vi "test_Export Configuration_Error.vi"(8 "error in (no error)":errorcluster, 11 "TestCase in":refnum<class "FPGA Addon Scripting API Unit Tests.lvclass">=refnum) -> (0 "error out":errorcluster, 3 "TestCase out":refnum<class "FPGA Addon Scripting API Unit Tests.lvclass">)   [LabVIEW 2026, in "FPGA Addon Scripting API Unit Tests.lvclass"]
uses:
  FPGA Addon Scripting API Unit Tests.lvclass
  FPGA Addon Test Class/FPGA Addon Test Class.lvclass
  APIs/Scripting API/Scripting API.lvlib
  APIs/Scripting API/Public/Bitfile Resources/Import Bitfile Scalars (Instances)/Import Scalars - all.vi
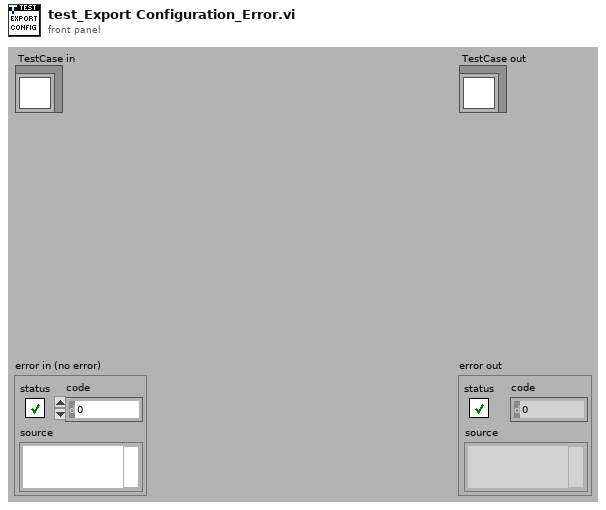
[diagram p1: front panel]
types:
  T1 = typedef "Custom Device API.lvlib/Custom Device Item Ref.ctl" = u64
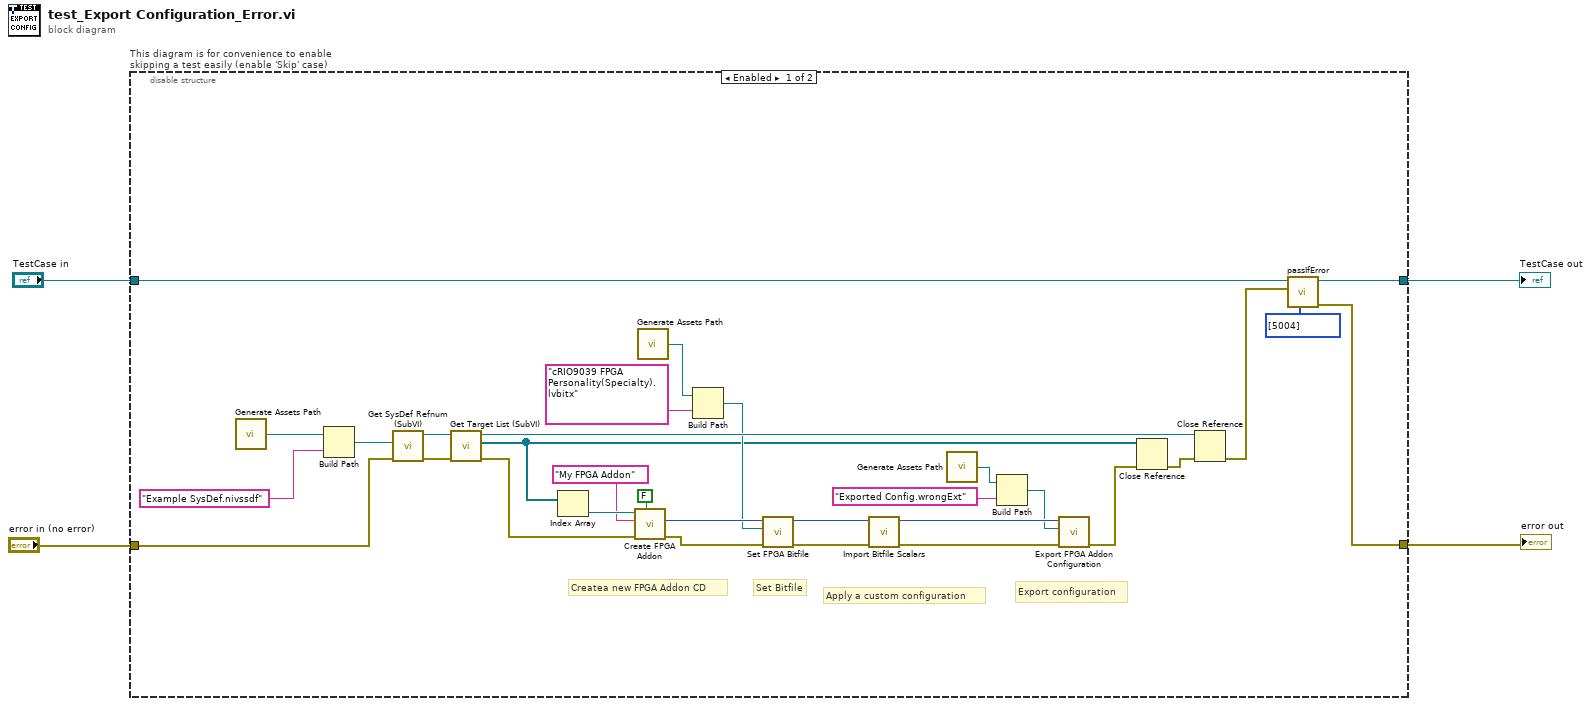
[diagram p0: block diagram]
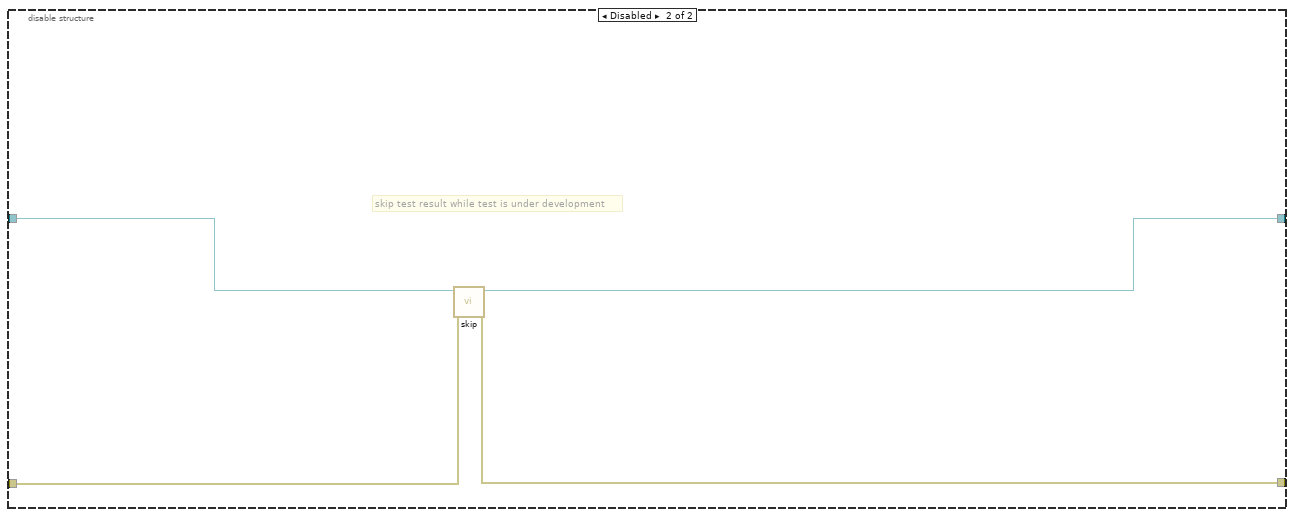
[diagram p2: hidden frame]
diagram:
  n1 = disable-structure "This diagram is for convenience to enable skipping a test easily (enable 'Skip' case)" shown="Enabled" {
    disable-tunnel: "TestCase in" -> [w9 w39]
    disable-tunnel: [w6 w37] -> w1
    disable-tunnel: [w7 w38] -> w3
    disable-tunnel: "error in (no error)" -> [w29 w36]
    frame Enabled {
      # "Export configuration"
      # "Apply a custom configuration"
      # "Set Bitfile"
      # "Createa new FPGA Addon CD"
      n2 = call "Generate Assets Path.vi"() -> ("Assets path"=w35:path)
      n3 = Build Path(base path=w35, name or relative path="Example SysDef.nivssdf") -> (appended path=w33:path)
      n4 = call "Get SysDef Refnum (SubVI).vi"("error in (no error)"=w29, "System Definition path"=w33) -> ("error out"=w28:errorcluster, "NationalInstruments.VeriStand.SystemDefinitionAPI.SystemDefinition"=w32:refnum<k39>)  [unwired: 8 in]
      n5 = call "Get Target List (SubVI).vi"("error in (no error)"=w28, "NationalInstruments.VeriStand.SystemDefinitionAPI.SystemDefinition"=w32) -> ("error out"=w27:errorcluster, "Target List Refnums"=w12:refnum<k39>[], "NationalInstruments.VeriStand.SystemDefinitionAPI.SystemDefinition"=w26:refnum<k39>)  [unwired: 7 in]
      n6 = Index Array(array=w12) -> (element=w31:refnum<k39>)  [unwired: 1 in]
      n7 = call "Create FPGA Addon.vi"("group scalars"=FALSE, "error in"=w27, "FPGA addon name"="My FPGA Addon", "NationalInstruments.VeriStand.SystemDefinitionAPI.Target"=w31) -> ("error out"=w13:errorcluster, "FPGA addon refnum"=w23:T1)  [unwired: 5 in, 1 out]
      n8 = call "Generate Assets Path.vi"() -> ("Assets path"=w22:path)
      n9 = Build Path(base path=w22, name or relative path="cRIO9039 FPGA Personality(Specialty).lvbitx") -> (appended path=w20:path)
      n10 = call "Set FPGA Bitfile.vi"("error in"=w13, "FPGA bitfile path"=w20, "FPGA addon refnum in"=w23) -> ("error out"=w19:errorcluster, "FPGA addon refnum out"=w18:T1)  [unwired: 7 in]
      n11 = call-poly "Import Bitfile Scalars.vi"("error in"=w19, "FPGA addon refnum in"=w18) -> ("error out"=w17:errorcluster, "FPGA addon refnum out"=w16:T1)  [unwired: 7 in, 1 out]
      n12 = call "Generate Assets Path.vi"() -> ("Assets path"=w15:path)
      n13 = Build Path(base path=w15, name or relative path="Exported Config.wrongExt") -> (appended path=w11:path)
      n14 = call "Export FPGA Addon Configuration.vi"("error in"=w17, "export file path"=w11, "FPGA addon refnum in"=w16) -> ("error out"=w10:errorcluster)  [unwired: 7 in, 1 out]
      n15 = Close Reference(reference=w12, error in (no error)=w10) -> (error out=w25:errorcluster)
      n16 = Close Reference(reference=w26, error in (no error)=w25) -> (error out=w8:errorcluster)
      n17 = call-dynamic "passIfError.vi"("passing error codes (default = any error code)"=i32[] [5004], "error"=w8, "TestCase in"=w9) -> ("error out"=w7:errorcluster, "TestCase out"=w6:refnum<class "FPGA Addon Scripting API Unit Tests.lvclass">)  [unwired: 7 in]
    }
    frame Disabled {
      # "skip test result while test is under development"
      n18 = call <vilib>:"skip.vi"("error in (no error)"=w36, "TestCase in"=w39) -> ("error out"=w38:errorcluster, "TestCase out"=w37:refnum<class "FPGA Addon Scripting API Unit Tests.lvclass">)  [unwired: 8 in]
    }
  }
  "error out" <- w3
  "TestCase out" <- w1
